vi "send_outlook_mail_activex[1].vi"(4 "BCC":string, 5 "Attachement":path, 6 "CC":string, 7 "Importance":i32(ring)=1 items=["Low", "Normal", "High"], 8 "error in":errorcluster, 9 "Message":string, 10 "Subject":string, 11 "To":string) -> (0 "error out":errorcluster)   [LabVIEW 2013]
doc: "This example uses Microsoft Outlook activeX objects to create a new message and then send that message using the Microsoft Outlook engine. The VI was developed and testing using Microsoft Outlook 2002, but most version of Microsoft Outlook should be compatible with the program.\n\nEnter data into the To, Subject, and message controls on the front panel. The other controls, CC and BCC, are optional. When using multiple email addresses separate addresses with a semicolon. \n\nRun the VI to send an email to the specified email address. If you have the E-mail security update installed with Microsoft Outlook 2002, you will be prompted to authorize the automated email and override the security warning. Click OK in the message box to send the email.\n\nNote: \nFor truly automated messaging, you can override this warning message programmatically using third party software."
panel:
  in  "Outlook._MailItem":refnum<k7>
  in  "Outlook._Application":refnum<k7>
  # "Select Help»Show Context Help and move the cursor over the VI icon to display help for this VI."
  # "Sending E-Mail with MS Outlook Using ActiveX"
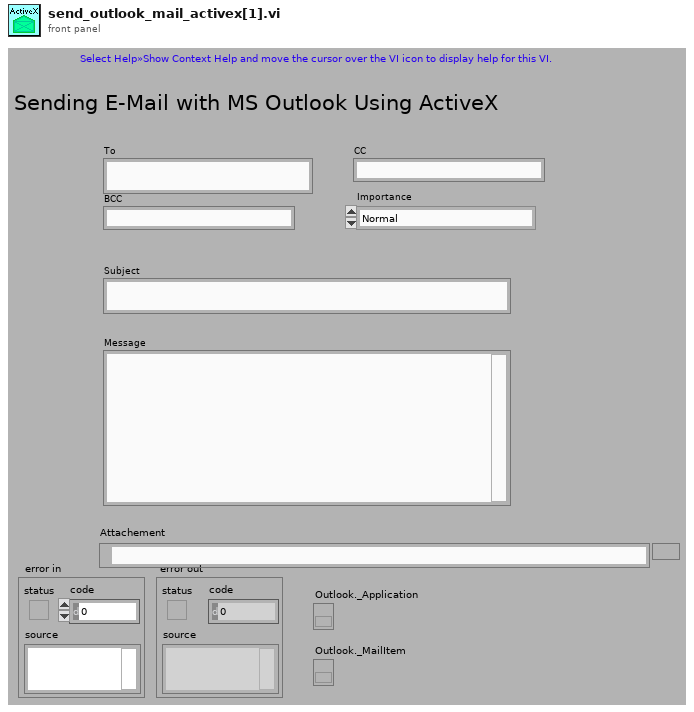
[diagram p1: front panel]
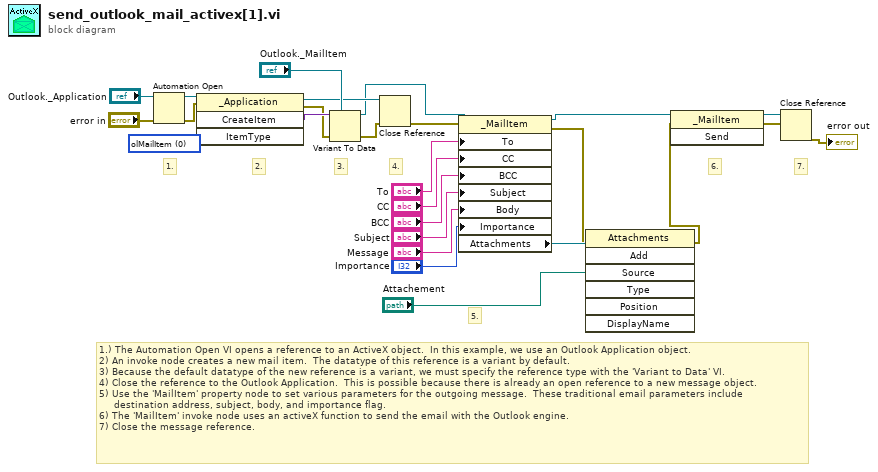
[diagram p0: block diagram]
diagram:
  w24 = 0 items=["olMailItem", "olAppointmentItem", "olContactItem", "olTaskItem", "olJournalItem", "olNoteItem", "olPostItem"] ("ItemType")
  # "7."
  # "1.) The Automation Open VI opens a reference to an ActiveX object.  In this example, we use an Outlook Application object.\n2) An invoke node creates a new mail item.  The datatype of this reference is a variant by default.\n3) Because the default datatype of the new reference is a variant, we must specify the reference type with the 'Variant to Data' VI.\n4) Close the reference to the Outlook Application.  This is possible because there is already an open reference to a new message object.\n5) Use the 'MailItem' property node to set various parameters for the outgoing message.  These traditional email parameters include\n     destination address, subject, body, and importance flag.\n6) The 'MailItem' invoke node uses an activeX function to send the email with the Outlook engine.\n7) Close the message reference."
  # "6."
  # "5."
  # "4."
  # "3."
  # "2."
  # "1."
  n1 = Automation Open(error in (no error)="error in", Automation Refnum="Outlook._Application") -> (Automation Refnum=w25:refnum<k7>, error out=w15:errorcluster)  [unwired: 2 in]
  n2 = invoke class="_Application" method="CreateItem"(reference=w25, error in=w15, "ItemType"=w24) -> (reference out=w19:refnum<k7>, error out=w13:errorcluster, "CreateItem"=w23:variant)  [unwired: 1 in, 1 out]
  n3 = Variant To Data(error in=w13, type="Outlook._MailItem", Variant=w23) -> (data=w18:refnum<k7>, error out=w12:errorcluster)
  n4 = Close Reference(reference=w19, error in (no error)=w12) -> (error out=w11:errorcluster)
  n5 = property class="_MailItem"(reference=w18, error in=w11, "To"="To", "CC"="CC", "BCC"="BCC", "Subject"="Subject", "Body"="Message", "Importance"="Importance") -> (reference out=w21:refnum<k7>, error out=w1:errorcluster, "Attachments"=w4:refnum<k7>)
  n6 = invoke class="Attachments" method="Add"(reference=w4, error in=w1, "Source"="Attachement") -> (error out=w2:errorcluster)  [unwired: 4 in, 6 out]
  n7 = invoke class="_MailItem" method="Send"(reference=w21, error in=w2) -> (reference out=w17:refnum<k7>, error out=w16:errorcluster)  [unwired: 1 in, 1 out]
  n8 = Close Reference(reference=w17, error in (no error)=w16) -> (error out=→"error out":errorcluster)
